vi "GUI_PI_Stages.vi"() -> ()   [LabVIEW 2013]
uses:
  <vilib>/Utility/tcp.llb/UDP Multicast Write-Only Open.vi
  <vilib>/Utility/file.llb/Read From Spreadsheet File (string).vi
panel:
  in  "QuadPosXYZ 2":dbl[](array[numeric])=[-4.0, 0.604, -0.05]
  out "Q2 controls":refnum<vi>[](array[refnum])
  out "Q1 controls":refnum<vi>[](array[refnum])
  out "DataSocket\nconnected":bool=TRUE
  out "QuadPosXYZ":dbl[](array[numeric])=[2.95001, 1.21, 2.60006, 2.57018, 2.80001, 11.9001]
  in  "Device Name 2":string="QuadZ"
  in  "Device Name":string="QuadXY"
  out "shotnumber":i32=-1
  out "con ref array":refnum<vi>[](array[refnum])
  out "MC Multicast":refnum<k16>
  out "new Slow Data":bool
  out "new Device Data":bool
  in  "Tab Control":T1(tab)
  out "limit Z2 (-)":dbl=-4.19999 format="%#_6f"
  out "limit Z1 (-)":dbl=-2.0 format="%#_6f"
  out "limit Z2 (+)":dbl=17.1 format="%#_6f"
  out "limit Z1 (+)":dbl=18.900100000000002 format="%#_6f"
  out "Z1":dbl=2.80001 format="%#_6f"
  in  "Q2 Z+":bool
  in  "Q2 Z-":bool
  out "Z2":dbl=11.9001 format="%#_6f"
  in  "Q1 Z+":bool
  in  "Q1 Z-":bool
  in  "Q2 Y+":bool
  in  "Q2 Y-":bool
  in  "Q2 X+":bool
  in  "Q2 X-":bool
  in  "Q1 Y-":bool
  in  "Q1 X+":bool
  in  "Q1 X-":bool
  in  "halt!":bool
  out "Y1":dbl=2.60006 format="%#_6f"
  out "Y2":dbl=2.57018 format="%#_6f"
  out "X1":dbl=2.95001 format="%#_6f"
  out "X2":dbl=1.21 format="%#_6f"
  out "error message":string
  out "error":bool
  in  "moving1":bool
  in  "moving2":bool
  in  "moving3":bool
  in  "moving4":bool
  out "Moving":bool
  out "Moving":bool
  in  "neglimit 1":bool
  in  "neglimit 2":bool
  in  "neglimit 3":bool
  in  "neglimit 4":bool
  in  "poslimit 1":bool
  in  "poslimit 3":bool
  in  "poslimit 4":bool
  in  "poslimit 2":bool
  in  "Q1 Y+":bool
  in  "Moving":bool
  in  "Moving":bool
  in  "poslimit 6":bool
  in  "neglimit 6":bool
  in  "poslimit 5":bool
  in  "neglimit 5":bool
  in  "servostatus 6":bool
  in  "servostatus 5":bool
  in  "servostatus 4":bool
  in  "servostatus 2":bool
  in  "servostatus 3":bool
  in  "servostatus 1":bool
  in  "save mode 2":bool=TRUE
  in  "save mode 3":bool=TRUE
  in  "setSaveMode":bool=TRUE
  in  "StepSize":dbl=1.5 format="%#_6f"
  out "data con closed":bool=TRUE
  out "data\nconnection 2":bool
  out "data con closed 2":bool=TRUE
  out "data\nconnection 3":bool
  out "Hexapos (Z)":dbl=-4.0
  out "D1":dbl=37.000009999999996 format="%#_6f"
  out "D2":dbl=24.70009 format="%#_6f"
  out "In Range?":bool=TRUE
  out "In Range?":bool=TRUE
  in  "Remote Host 2":string="192.168.10.75"
  in  "port or service name 2":u16=65534
  out "local Port":u16=65000
  out "Remote Host":string="192.168.10.73"
  out "port or service name":u16=65535
  in  "timeout ms (100)":i32=20
  in  "Multicast":bool
  out "#shot":i32
  in  "String 2":string
  in  "send CMD":bool
  in  "reset":bool
  in  "New Shot":bool
  in  "Data String 2":string="scalar>>pos2,2.800010\r\npos4,11.900100\r\nmoving2,off\r\nmoving4,off\r\ncloseaftermove,on\r\nservostatus2,off\r\nservostatus4,off\r\nneglimit2,off\r\nneglimit4,off\r\nposlimit2,off\r\nposlimit4,off\r\n"
  out "fast ID":refnum<k16>
  out "slow ID":refnum<k16>
  out "data connection ID":refnum<k5>
  out "connections":variant[](array[variant])=[variant(refnum<k16> refnum), variant(refnum<k16> refnum)]
  in  "time to wait":i32=25
  in  "Subscriber list 2":string="wait>>pos1,pos2,pos3,pos4,moving1,moving2,moving3,moving4,closeaftermove,servostatus1,servostatus2,servostatus3,servostatus4,neglimit1,neglimit2,neglimit3,neglimit4,poslimit1,poslimit2,poslimit3,poslimit4"
  in  "Data String":string="scalar>>pos1,2.950010\r\npos2,1.210000\r\npos3,2.600060\r\npos4,2.570180\r\nmoving1,off\r\nmoving2,off\r\nmoving3,off\r\nmoving4,off\r\ncloseaftermove,on\r\nservostatus1,off\r\nservostatus2,off\r\nservostatus3,off\r\nservostatus4,off\r\nneglimit1,off\r\nneglimit2,off\r\nneglimit3,off\r\nneglimit4,off\r\nposlimit1,off\r\nposlimit2,off\r\nposlimit3,off\r\nposlimit4,off\r\n"
  out "data connection ID 2":refnum<k5>
  in  "Subscriber list 3":string="wait>>pos2,pos4,moving2,moving4,closeaftermove,servostatus2,servostatus4,neglimit2,neglimit4,poslimit2,poslimit4"
  out "all rows":string[][](array[string])=[["localport", "65000"], ["port", "65535"], ["remotehost", "192.168.10.73"]]
  out "path":path=path "X:/Software/LOASIS Control System/Developers Version/Interface/GUI_PI_Stages/192.168.10.157.txt"
  out "My IP":string="192.168.10.157"
  out "error out":errorcluster
  in  "stop":bool
  # "QUAD 1"
  # "QUAD 2"
  # "connected"
  # "connected"
  # "Servo \nStatus"
  # "XY"
  # "Z"
  # "61525"
  # "65535"
  # "61533"
  # "localhost"
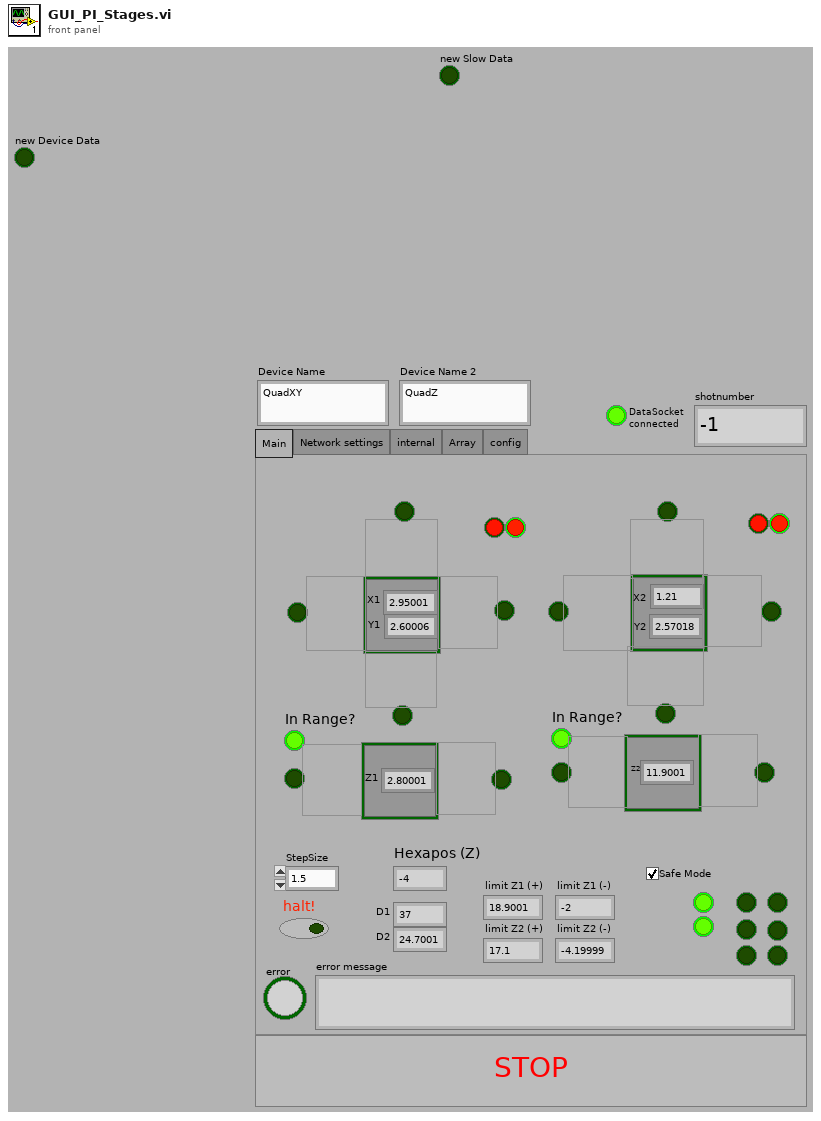
[diagram p1: front panel]
types:
  T1 = enum32{"Main", "Network settings", "internal", "Array", "config"}
  T2 = typedef "LVDataSocketStatusTypeDef.ctl" = cluster{"Code":enum32{"Invalid Status", "Unconnected", "Active", "Idle", "Error", "Connecting"}, "Text":string}
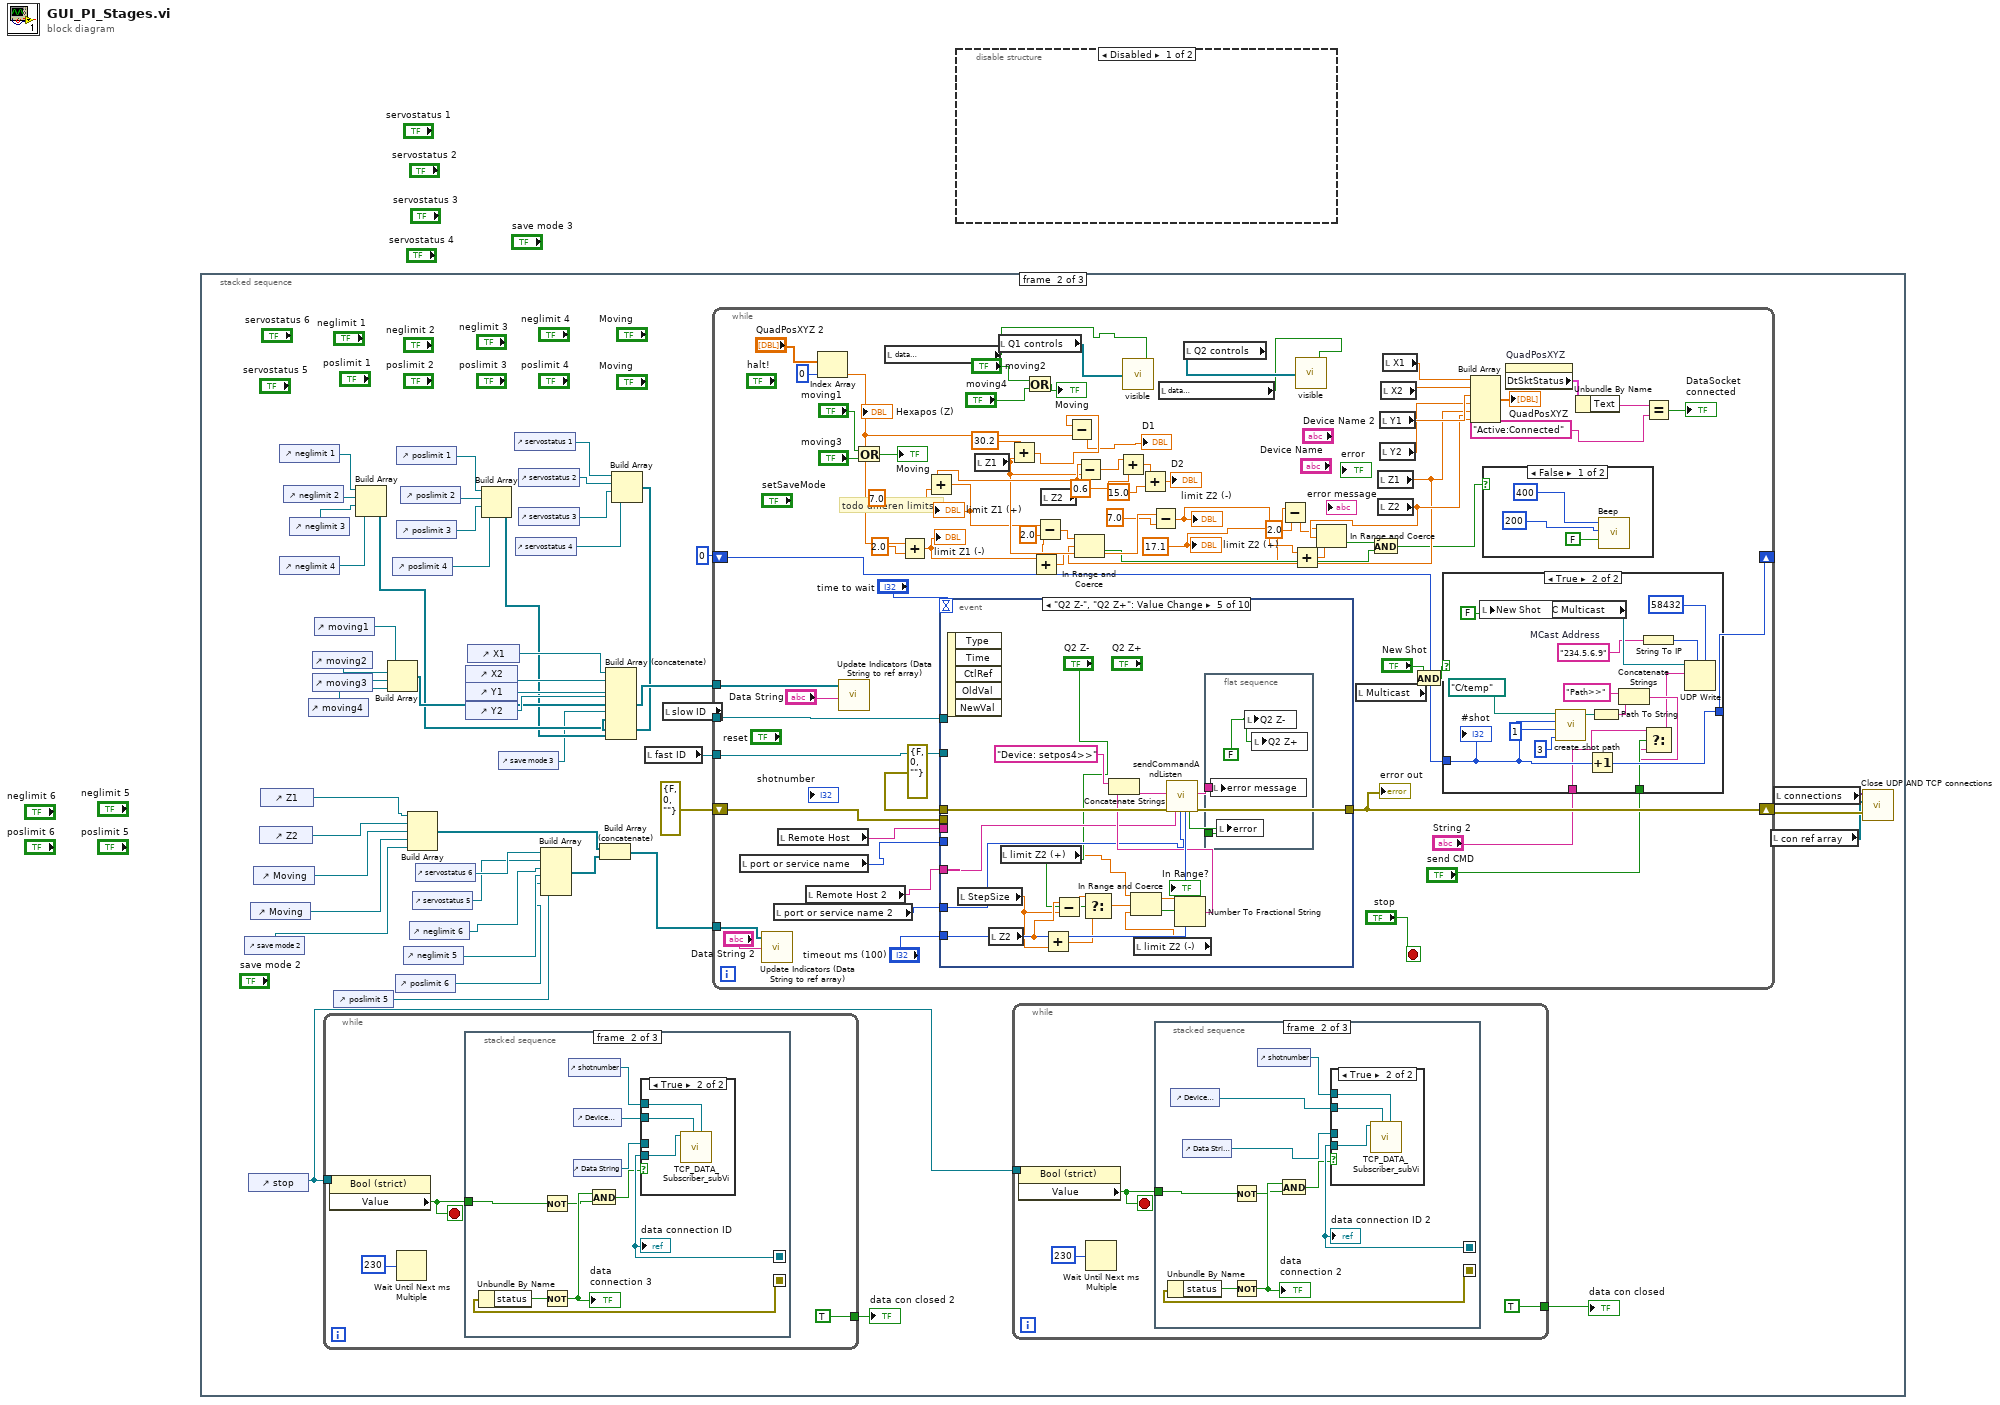
[diagram p0: block diagram]
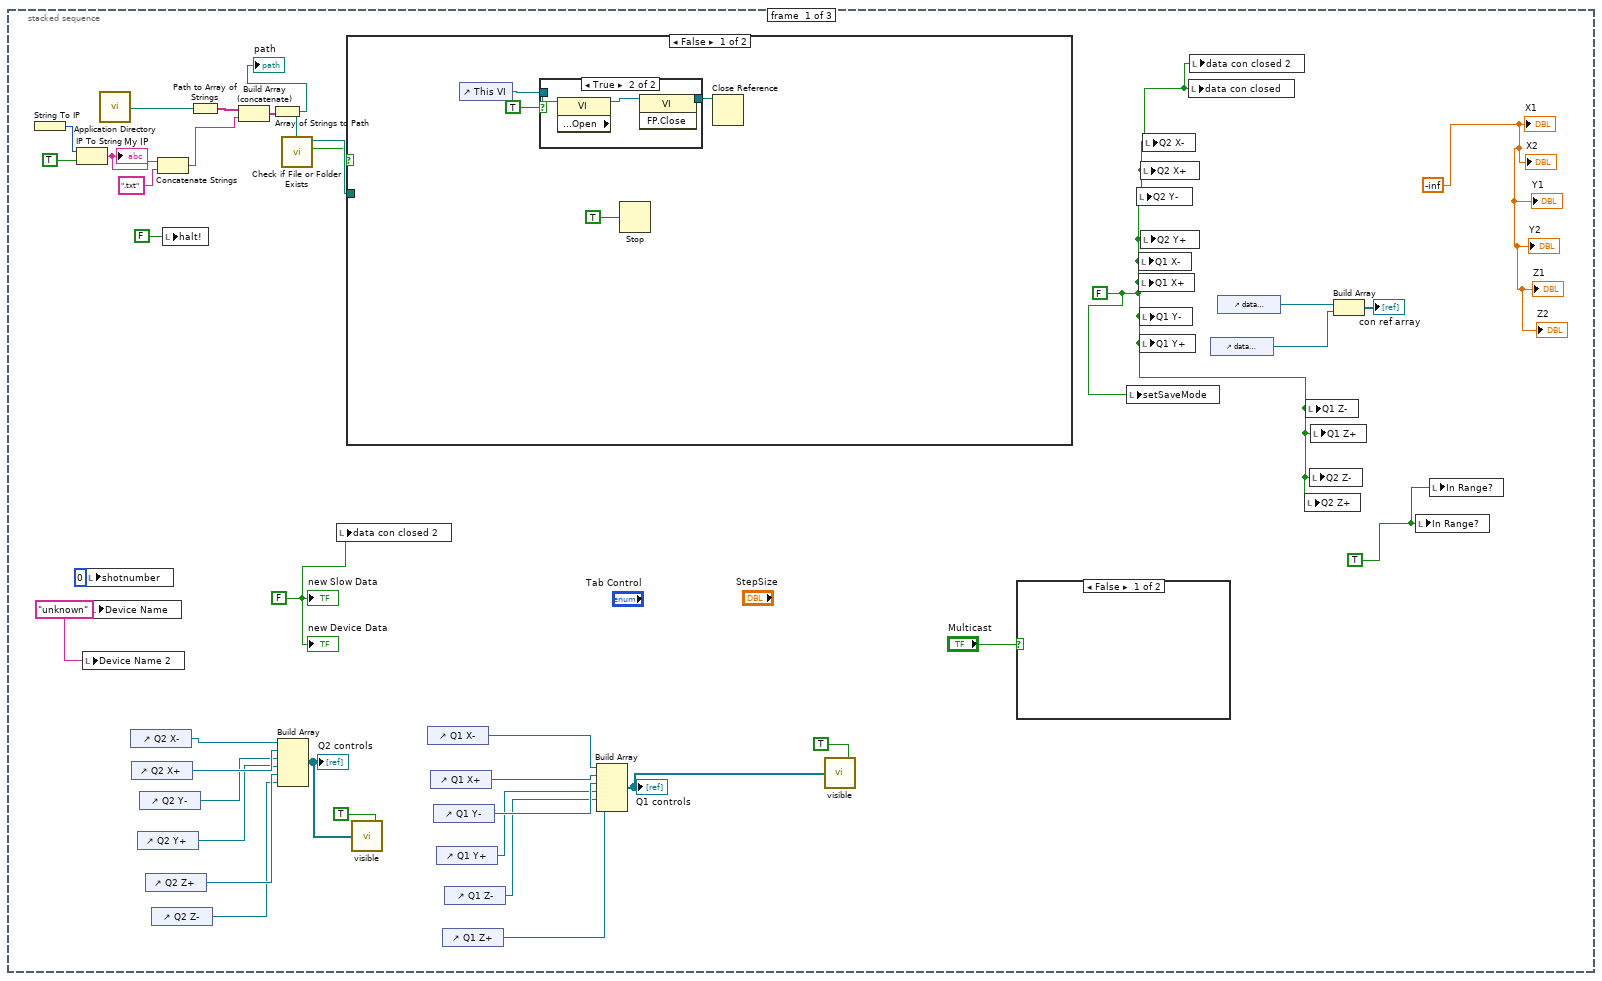
[diagram p3: hidden frame]
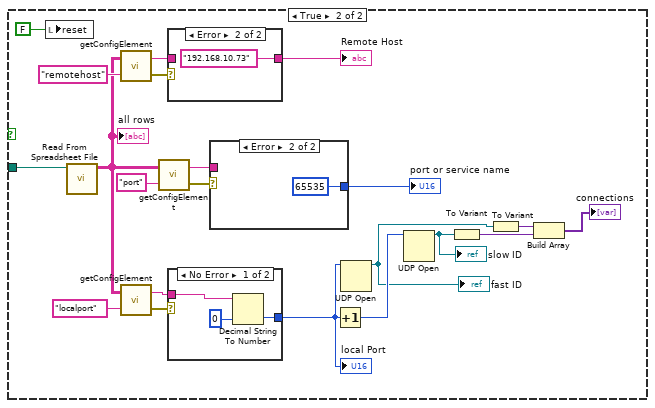
[diagram p5: hidden frame]
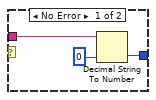
[diagram p6: hidden frame]
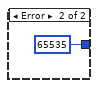
[diagram p8: hidden frame]
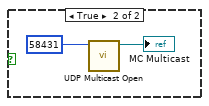
[diagram p9: hidden frame]
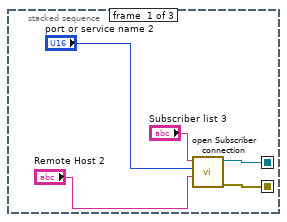
[diagram p10: hidden frame]
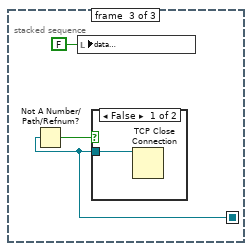
[diagram p12: hidden frame]
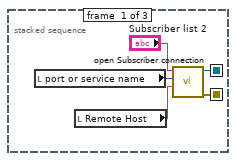
[diagram p14: hidden frame]
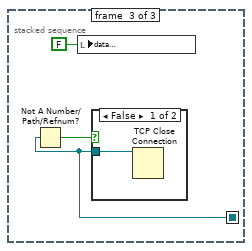
[diagram p16: hidden frame]
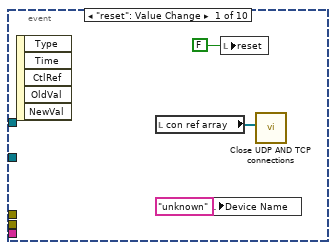
[diagram p20: hidden frame]
diagram:
  n1 = stacked-sequence {
    frame #0 {
      w1 = TRUE ("Q1 X-")
      w19 = -inf
      w18 = FALSE ("Q1 X-")
      w20 = "unknown" ("Device Name")
      w23 = FALSE ("new Device Data")
      n2 = String To IP() -> (0:w32:u32)  [unwired: 1 in]
      n3 = IP To String(1:TRUE ("dot notation? (F)"), 2:w32) -> (0:w30:string)
      "My IP" <- w30
      n4 = local write "Device Name 2"(w20) -> ()
      n5 = local write "shotnumber"(0 ("shotnumber")) -> ()
      n6 = local write "Device Name"(w20) -> ()
      n7 = call <vilib>:"Application Directory.vi"() -> ("Application Directory"=w28:path)
      n8 = control-ref of="Q2 X-"() -> (w17:refnum<vi>)
      n9 = control-ref of="Q2 X+"() -> (w16:refnum<vi>)
      n10 = control-ref of="Q2 Y+"() -> (w14:refnum<vi>)
      n11 = control-ref of="Q2 Y-"() -> (w15:refnum<vi>)
      n12 = control-ref of="Q2 Z+"() -> (w13:refnum<vi>)
      n13 = control-ref of="Q2 Z-"() -> (w12:refnum<vi>)
      n14 = Concatenate Strings(w30, ".txt" ("pattern")) -> (w27:string)
      n15 = local write "halt!"(FALSE ("halt!")) -> ()
      n16 = Path to Array of Strings(0:w28) -> (2:w34:string[])  [unwired: 1 out]
      n17 = Build Array (concatenate)(w34, w27) -> (w33:string[])
      n18 = Array of Strings to Path(0:w33) -> (2:w26:path)  [unwired: 1 in]
      "path" <- w26
      n19 = Build Array(w17, w16, w15, w14, w13, w12) -> (w3:refnum<vi>[])
      "Q2 controls" <- w3
      n20 = call <vilib>:"Check if File or Folder Exists.vi"("path"=w26) -> ("file or folder exists?"=w24:bool, "dup path"=w25:path)  [unwired: 8 in, 1 out]
      n21 = local write "data con closed 2"(w23) -> ()
      n22 = case shown="False" w24 {
        tunnel: w25 -> [_ w49]
        frame False {
          n23 = control-ref of="This VI"() -> (w41:refnum<vi>)
          n24 = case shown="True" TRUE {
            tunnel: w41 -> [w43 w46]
            tunnel: [w43 w44] -> w40
            frame False {
            }
            frame True {
              n25 = property class="VI" props=["Front Panel.Open"](reference=w46) -> (reference out=w45:refnum<vi>)  [unwired: 1 in, 2 out]
              n26 = invoke class="VI" method="FP.Close"(reference=w45) -> (reference out=w44:refnum<vi>)  [unwired: 2 in, 2 out]
            }
          }
          n27 = Stop(stop? (T)=TRUE) -> ()
          n28 = Close Reference(reference=w40) -> ()  [unwired: 1 in, 1 out]
        }
        frame True {
          n29 = local write "reset"(FALSE ("reset")) -> ()
          n30 = call-poly <vilib>:"Read From Spreadsheet File.vi"("file path (dialog if empty)"=w49) -> ("all rows"=w51:string[][])  [unwired: 6 in, 4 out]
          "all rows" <- w51
          n31 = call "getConfigElement.vi"("element"="remotehost", "all rows"=w51) -> ("error in"=w48:errorcluster, "value"=w56:string)
          n32 = call "getConfigElement.vi"("element"="localport", "all rows"=w51) -> ("error in"=w58:errorcluster, "value"=w59:string)
          n33 = call "getConfigElement.vi"("element"="port", "all rows"=w51) -> ("error in"=w47:errorcluster, "value"=w53:string)
          n34 = case shown="Error" w48 {
            tunnel: w56 -> [w72 _]
            tunnel: [w72 "192.168.10.73" ("value")] -> w54
            frame No Error {
            }
            frame Error {
            }
          }
          "Remote Host" <- w54
          n35 = case shown="No Error" w58 {
            tunnel: w59 -> [w76 _]
            tunnel: [w74 u16 65535] -> w57
            frame No Error {
              n36 = Decimal String To Number(string=w76, default (0L)=u16 0 ("local Port")) -> (number=w74:u16)  [unwired: 1 in, 1 out]
            }
            frame Error {
            }
          }
          "local Port" <- w57
          n37 = case shown="Error" w47 {
            tunnel: w53 -> [w70 _]
            tunnel: [w68 u16 65535] -> w50
            frame No Error {
              n38 = Decimal String To Number(string=w70, default (0L)=u16 0 ("local Port")) -> (number=w68:u16)  [unwired: 1 in, 1 out]
            }
            frame Error {
            }
          }
          "port or service name" <- w50
          n39 = Increment(x=w57) -> (x+1=w67:u16)
          n40 = UDP Open(11:w57) -> (port=w65:refnum<k16>)  [unwired: 4 in, 2 out]
          "fast ID" <- w65
          n41 = UDP Open(11:w67) -> (port=w64:refnum<k16>)  [unwired: 4 in, 2 out]
          "slow ID" <- w64
          n42 = To Variant(anything=w64) -> (Variant=w62:variant)
          n43 = To Variant(anything=w65) -> (Variant=w63:variant)
          n44 = Build Array(w63, w62) -> (→"connections":variant[])
        }
      }
      n45 = call "visible.vi"("visible"=TRUE, "Array"=w3) -> ()
      n46 = control-ref of="Q1 X-"() -> (w11:refnum<vi>)
      n47 = control-ref of="Q1 X+"() -> (w10:refnum<vi>)
      n48 = control-ref of="Q1 Y-"() -> (w9:refnum<vi>)
      n49 = control-ref of="Q1 Y+"() -> (w8:refnum<vi>)
      n50 = control-ref of="Q1 Z+"() -> (w6:refnum<vi>)
      n51 = control-ref of="Q1 Z-"() -> (w7:refnum<vi>)
      n52 = Build Array(w11, w10, w9, w8, w7, w6) -> (w5:refnum<vi>[])
      "Q1 controls" <- w5
      n53 = call "visible.vi"("visible"=TRUE, "Array"=w5) -> ()
      n54 = case shown="False" "Multicast" {
        frame False {
        }
        frame True {
          n55 = call-poly <vilib>:"UDP Multicast Open.vi"("port"=u16 58431) -> ("connection ID"=→"MC Multicast":refnum<k16>)  [unwired: 9 in, 1 out]
        }
      }
      n56 = local write "setSaveMode"(w18) -> ()
      n57 = local write "Q2 Y-"(w18) -> ()
      n58 = local write "Q1 X-"(w18) -> ()
      n59 = local write "Q1 X+"(w18) -> ()
      n60 = local write "Q1 Y-"(w18) -> ()
      n61 = local write "Q1 Y+"(w18) -> ()
      n62 = local write "Q2 X+"(w18) -> ()
      n63 = local write "Q2 Y+"(w18) -> ()
      n64 = local write "Q2 X-"(w18) -> ()
      n65 = local write "data con closed"(w18) -> ()
      n66 = local write "data con closed 2"(w18) -> ()
      n67 = control-ref of="data connection ID 2"() -> (w21:refnum<vi>)
      n68 = control-ref of="data connection ID"() -> (w38:refnum<vi>)
      n69 = local write "Q2 Z+"(w18) -> ()
      n70 = local write "Q1 Z-"(w18) -> ()
      n71 = local write "Q2 Z-"(w18) -> ()
      n72 = local write "Q1 Z+"(w18) -> ()
      n73 = Build Array(w38, w21) -> (→"con ref array":refnum<vi>[])
      n74 = local write "In Range?"(w1) -> ()
      n75 = local write "In Range?"(w1) -> ()
      "new Device Data" <- w23
      "new Slow Data" <- w23
      "X1" <- w19
      "X2" <- w19
      "Y2" <- w19
      "Y1" <- w19
      "Z1" <- w19
      "Z2" <- w19
    }
    frame #1 {
      n76 = control-ref of="save mode 2"() -> (w90:refnum<vi>)
      n77 = control-ref of="stop"() -> (w96:refnum<vi>)
      n78 = control-ref of="Moving"() -> (w91:refnum<vi>)
      n79 = control-ref of="Moving"() -> (w92:refnum<vi>)
      n80 = control-ref of="Z2"() -> (w93:refnum<vi>)
      n81 = control-ref of="Z1"() -> (w94:refnum<vi>)
      n82 = control-ref of="neglimit 1"() -> (w107:refnum<vi>)
      n83 = control-ref of="neglimit 4"() -> (w104:refnum<vi>)
      n84 = control-ref of="neglimit 2"() -> (w106:refnum<vi>)
      n85 = control-ref of="neglimit 3"() -> (w105:refnum<vi>)
      n86 = control-ref of="moving4"() -> (w114:refnum<vi>)
      n87 = control-ref of="moving2"() -> (w116:refnum<vi>)
      n88 = control-ref of="moving3"() -> (w115:refnum<vi>)
      n89 = control-ref of="moving1"() -> (w117:refnum<vi>)
      n90 = while {
        tunnel: [TRUE] -> w97
        tunnel: w96 -> [w157]
        stop <- w156 stop-if-true
        n91 = property class="Bool (strict)"(reference=w157) -> ("Value"=w156:bool)  [unwired: 1 in, 2 out]
        n92 = Wait Until Next ms Multiple(millisecond multiple=u32 230) -> ()  [unwired: 1 out]
        n93 = stacked-sequence {
          seq-local: [w161 _ _] -> [_ w173 w179]
          seq-local: [w160 _ _] -> [_ w172 _]
          tunnel: w156 -> [_ w166 _]
          frame #0 {
            n94 = local read "port or service name"() -> (w163:u16)
            n95 = local read "Remote Host"() -> (w162:string)
            n96 = call "open Subscriber connection.vi"("Machine"=w162, "Port"=w163, "Subscriber list"="Subscriber list 2") -> ("error out"=w160:errorcluster, "connection ID"=w161:refnum<k5>)  [unwired: 3 in]
          }
          frame #1 {
            n97 = Unbundle By Name(w172) -> ("status"=w169:bool)
            n98 = Not(x=w166) -> (.not. x?=w167:bool)
            n99 = Not(x=w169) -> (.not. x?=w168:bool)
            "data\nconnection 3" <- w168
            n100 = control-ref of="shotnumber"() -> (w171:refnum<vi>)
            n101 = control-ref of="Device Name"() -> (w170:refnum<vi>)
            n102 = control-ref of="Data String"() -> (w174:refnum<vi>)
            n103 = And(x=w168, y=w167) -> (x .and. y?=w165:bool)
            n104 = case shown="True" w165 {
              tunnel: w174 -> [_ _]
              tunnel: w173 -> [_ w175]
              tunnel: w171 -> [_ w177]
              tunnel: w170 -> [_ w176]
              frame False {
              }
              frame True {
                n105 = call "TCP_DATA_Subscriber_subVi.vi"("shot number"=w177, "whatamI"=w176, "connection ID"=w175) -> ()  [unwired: 8 in, 1 out]
              }
            }
            "data connection ID" <- w173
          }
          frame #2 {
            n106 = Not A Number/Path/Refnum?(number/path/refnum=w179) -> (NaN/Path/Refnum?=w180:bool)
            n107 = local write "data\nconnection 3"(FALSE ("status 2")) -> ()
            n108 = case shown="False" w180 {
              tunnel: w179 -> [w181 _]
              frame False {
                n109 = TCP Close Connection(connection ID=w181) -> ()  [unwired: 2 in, 2 out]
              }
              frame True {
              }
            }
          }
        }
      }
      "data con closed 2" <- w97
      n110 = control-ref of="poslimit 5"() -> (w84:refnum<vi>)
      n111 = Build Array(w107, w106, w105, w104) -> (w99:refnum<vi>[])
      n112 = Build Array(w117, w116, w115, w114) -> (w113:refnum<vi>[])
      n113 = control-ref of="poslimit 4"() -> (w100:refnum<vi>)
      n114 = control-ref of="poslimit 6"() -> (w85:refnum<vi>)
      n115 = control-ref of="poslimit 1"() -> (w103:refnum<vi>)
      n116 = control-ref of="poslimit 3"() -> (w101:refnum<vi>)
      n117 = control-ref of="poslimit 2"() -> (w102:refnum<vi>)
      n118 = control-ref of="neglimit 5"() -> (w86:refnum<vi>)
      n119 = Build Array(w94, w93, w92, w91, w90) -> (w83:refnum<vi>[])
      n120 = control-ref of="neglimit 6"() -> (w87:refnum<vi>)
      n121 = control-ref of="servostatus 5"() -> (w88:refnum<vi>)
      n122 = control-ref of="servostatus 6"() -> (w89:refnum<vi>)
      n123 = control-ref of="X2"() -> (w120:refnum<vi>)
      n124 = control-ref of="Y1"() -> (w119:refnum<vi>)
      n125 = control-ref of="Y2"() -> (w118:refnum<vi>)
      n126 = control-ref of="X1"() -> (w126:refnum<vi>)
      n127 = Build Array(w103, w102, w101, w100) -> (w98:refnum<vi>[])
      n128 = control-ref of="save mode 3"() -> (w80:refnum<vi>)
      n129 = control-ref of="servostatus 1"() -> (w112:refnum<vi>)
      n130 = control-ref of="servostatus 4"() -> (w109:refnum<vi>)
      n131 = control-ref of="servostatus 2"() -> (w111:refnum<vi>)
      n132 = control-ref of="servostatus 3"() -> (w110:refnum<vi>)
      n133 = Build Array(w89, w88, w87, w86, w85, w84) -> (w82:refnum<vi>[])
      n134 = Build Array (concatenate)(w83, w82) -> (w81:refnum<vi>[])
      n135 = Build Array(w112, w111, w110, w109) -> (w108:refnum<vi>[])
      n136 = Build Array (concatenate)(w126, w120, w119, w118, w113, w80, w108, w99, w98) -> (w124:refnum<vi>[])
      n137 = local read "fast ID"() -> (w128:refnum<k16>)
      n138 = local read "slow ID"() -> (w127:refnum<k16>)
      n139 = while {
        tunnel: w128 -> [w246]
        shift-right: [w244] -> w125
        shift-left: errorcluster {"status"=FALSE, "code"=0, "source"=""} ("error out") -> [w250]
        tunnel: w127 -> [w238]
        tunnel: w124 -> [w252]
        shift-right: [w243] -> _
        shift-left: 0 -> [w242]
        tunnel: w81 -> [w228]
        stop <- "stop" stop-if-true
        w186 = 2.0 ("y")
        w190 = 2.0 ("y")
        w192 = 17.1 ("y")
        # "todo differen limits"
        n140 = local read "port or service name"() -> (w247:u16)
        n141 = call "Update Indicators (Data String to ref array).vi"("Data String"="Data String 2", "Array"=w228) -> ()  [unwired: 4 in]
        n142 = local read "port or service name 2"() -> (w226:u16)
        n143 = local read "Remote Host"() -> (w248:string)
        n144 = local read "Remote Host 2"() -> (w227:string)
        n145 = Index Array(array="QuadPosXYZ 2", index=0) -> (element=w201:dbl)
        "Hexapos (Z)" <- w201
        n146 = call "Update Indicators (Data String to ref array).vi"("Data String"="Data String", "Array"=w252) -> ()  [unwired: 4 in]
        n147 = Or(x="moving1", y="moving3") -> (x .or. y?=→"Moving":bool)
        n148 = local read "data\nconnection 3"() -> (w214:bool)
        n149 = Add(x=w201, y=2.0) -> (x+y=w191:dbl)
        "limit Z1 (-)" <- w191
        n150 = event shown="[4] \"Q2 Z-\", \"Q2 Z+\": Value Change" {
          selector: _ -> [_ _ _ _ _ _ _ _ _ _]
          dyn-events: _ -> [_ _ _ _ _ _ _ _ _ _]
          timeout: "time to wait" -> [_ _ _ _ _ _ _ _ _ _]
          tunnel: w246 -> [_ _ _ _ _ _ _ _ _ _]
          tunnel: [_ w291 w310 w333 w356 w375 w394 w405 w422 w431] -> w244
          tunnel: errorcluster {"status"=FALSE, "code"=0, "source"=""} ("error out") -> [_ w292 w311 w334 w357 w376 w395 w415 w422 _]
          tunnel: w248 -> [_ w290 w309 _ _ w374 w393 w414 w429 _]
          tunnel: w247 -> [_ w289 w308 _ _ w373 w392 w413 w428 _]
          tunnel: "timeout ms (100)" -> [_ w288 w307 w332 w355 w372 w391 w401 _ _]
          tunnel: w238 -> [_ _ _ _ _ _ _ _ _ _]
          tunnel: w250 -> [_ _ _ _ _ _ _ _ _ w431]
          tunnel: w227 -> [_ _ _ w323 w347 _ _ w403 w419 _]
          tunnel: w226 -> [_ _ _ w324 w348 _ _ w402 w418 _]
          event "reset": Value Change {
            n151 = event-data() -> ()  [unwired: 1 in, 5 out]
            n152 = local read "con ref array"() -> (w277:refnum<vi>[])
            n153 = local write "Device Name"("unknown" ("Device Name")) -> ()
            n154 = local write "reset"(FALSE ("reset")) -> ()
            n155 = call "Close UDP AND TCP connections.vi"("appended array 2"=w277) -> ()  [unwired: 7 in]
          }
          event "Q1 X-", "Q1 X+": Value Change {
            n156 = event-data() -> ()  [unwired: 1 in, 5 out]
            n157 = local read "StepSize"() -> (w279:dbl)
            n158 = local read "X1"() -> (w280:dbl)
            n159 = Add(x=w280, y=w279) -> (x+y=w283:dbl)
            n160 = Subtract(x=w280, y=w279) -> (x-y=w284:dbl)
            n161 = Select(t=w284, s="Q1 X-", f=w283) -> (s? t:f=w282:dbl)
            n162 = Number To Fractional String(number=w282) -> (F-format string=w281:string)  [unwired: 3 in]
            n163 = Concatenate Strings("Device: setpos1>>" ("data in"), w281) -> (w293:string)
            n164 = call "sendCommandAndListen.vi"("command in"=w293, "error in"=w292, "Remote Host"=w290, "port or service name"=w289, "timeout ms (100)"=w288) -> ("error"=w286:bool, "error message"=w287:string, "error out"=w291:errorcluster)  [unwired: 7 in, 5 out]
            n165 = flat-sequence {
              tunnel: w287 -> [w297]
              tunnel: w286 -> [w296]
              frame #0 {
                w295 = FALSE ("Q1 X-")
                n166 = local write "error message"(w297) -> ()
                n167 = local write "error"(w296) -> ()
                n168 = local write "Q1 X+"(w295) -> ()
                n169 = local write "Q1 X-"(w295) -> ()
              }
            }
          }
          event "Q1 Y-", "Q1 Y+": Value Change {
            n170 = event-data() -> ()  [unwired: 1 in, 5 out]
            n171 = local read "StepSize"() -> (w299:dbl)
            n172 = local read "Y1"() -> (w300:dbl)
            n173 = Add(x=w300, y=w299) -> (x+y=w303:dbl)
            n174 = Subtract(x=w300, y=w299) -> (x-y=w304:dbl)
            n175 = Select(t=w304, s="Q1 Y-", f=w303) -> (s? t:f=w302:dbl)
            n176 = Number To Fractional String(number=w302) -> (F-format string=w301:string)  [unwired: 3 in]
            n177 = Concatenate Strings("Device: setpos3>>" ("data in"), w301) -> (w312:string)
            n178 = call "sendCommandAndListen.vi"("command in"=w312, "error in"=w311, "Remote Host"=w309, "port or service name"=w308, "timeout ms (100)"=w307) -> ("error"=w305:bool, "error message"=w306:string, "error out"=w310:errorcluster)  [unwired: 7 in, 5 out]
            n179 = flat-sequence {
              tunnel: w306 -> [w316]
              tunnel: w305 -> [w315]
              frame #0 {
                w314 = FALSE ("Q1 X-")
                n180 = local write "error message"(w316) -> ()
                n181 = local write "error"(w315) -> ()
                n182 = local write "Q1 Y+"(w314) -> ()
                n183 = local write "Q1 Y-"(w314) -> ()
              }
            }
          }
          event "Q1 Z-", "Q1 Z+": Value Change {
            n184 = event-data() -> ()  [unwired: 1 in, 5 out]
            n185 = local read "StepSize"() -> (w319:dbl)
            n186 = local read "Z1"() -> (w326:dbl)
            n187 = local read "limit Z1 (+)"() -> (w318:dbl)
            n188 = Add(x=w326, y=w319) -> (x+y=w328:dbl)
            n189 = Subtract(x=w326, y=w319) -> (x-y=w329:dbl)
            n190 = local read "limit Z1 (-)"() -> (w317:dbl)
            n191 = Select(t=w329, s="Q1 Z-", f=w328) -> (s? t:f=w322:dbl)
            n192 = In Range and Coerce(upper limit=w318, x=w322, lower limit=w317) -> (coerced(x)=w321:dbl, In Range?=→"In Range?":bool)
            n193 = Number To Fractional String(number=w321) -> (F-format string=w327:string)  [unwired: 3 in]
            n194 = Concatenate Strings("Device: setpos2>>" ("data in"), w327) -> (w335:string)
            n195 = call "sendCommandAndListen.vi"("command in"=w335, "error in"=w334, "Remote Host"=w323, "port or service name"=w324, "timeout ms (100)"=w332) -> ("error"=w330:bool, "error message"=w331:string, "error out"=w333:errorcluster)  [unwired: 7 in, 5 out]
            n196 = flat-sequence {
              tunnel: w331 -> [w339]
              tunnel: w330 -> [w338]
              frame #0 {
                w337 = FALSE ("Q1 X-")
                n197 = local write "error message"(w339) -> ()
                n198 = local write "error"(w338) -> ()
                n199 = local write "Q1 Z-"(w337) -> ()
                n200 = local write "Q1 Z+"(w337) -> ()
              }
            }
          }
          event "Q2 Z-", "Q2 Z+": Value Change {
            n201 = event-data() -> ()  [unwired: 1 in, 5 out]
            n202 = local read "StepSize"() -> (w342:dbl)
            n203 = local read "Z2"() -> (w349:dbl)
            n204 = local read "limit Z2 (+)"() -> (w341:dbl)
            n205 = Add(x=w349, y=w342) -> (x+y=w351:dbl)
            n206 = Subtract(x=w349, y=w342) -> (x-y=w352:dbl)
            n207 = Select(t=w352, s="Q2 Z-", f=w351) -> (s? t:f=w344:dbl)
            n208 = local read "limit Z2 (-)"() -> (w340:dbl)
            n209 = In Range and Coerce(upper limit=w341, x=w344, lower limit=w340) -> (coerced(x)=w345:dbl, In Range?=→"In Range?":bool)
            n210 = Number To Fractional String(number=w345) -> (F-format string=w350:string)  [unwired: 3 in]
            n211 = Concatenate Strings("Device: setpos4>>" ("data in"), w350) -> (w358:string)
            n212 = call "sendCommandAndListen.vi"("command in"=w358, "error in"=w357, "Remote Host"=w347, "port or service name"=w348, "timeout ms (100)"=w355) -> ("error"=w353:bool, "error message"=w354:string, "error out"=w356:errorcluster)  [unwired: 7 in, 5 out]
            n213 = flat-sequence {
              tunnel: w354 -> [w362]
              tunnel: w353 -> [w361]
              frame #0 {
                w360 = FALSE ("Q1 X-")
                n214 = local write "error message"(w362) -> ()
                n215 = local write "error"(w361) -> ()
                n216 = local write "Q2 Z-"(w360) -> ()
                n217 = local write "Q2 Z+"(w360) -> ()
              }
            }
          }
          event "Q2 Y-", "Q2 Y+": Value Change {
            n218 = event-data() -> ()  [unwired: 1 in, 5 out]
            n219 = local read "StepSize"() -> (w364:dbl)
            n220 = local read "Y2"() -> (w365:dbl)
            n221 = Add(x=w365, y=w364) -> (x+y=w368:dbl)
            n222 = Subtract(x=w365, y=w364) -> (x-y=w369:dbl)
            n223 = Select(t=w369, s="Q2 Y-", f=w368) -> (s? t:f=w367:dbl)
            n224 = Number To Fractional String(number=w367) -> (F-format string=w366:string)  [unwired: 3 in]
            n225 = Concatenate Strings("Device: setpos4>>" ("data in"), w366) -> (w377:string)
            n226 = call "sendCommandAndListen.vi"("command in"=w377, "error in"=w376, "Remote Host"=w374, "port or service name"=w373, "timeout ms (100)"=w372) -> ("error"=w370:bool, "error message"=w371:string, "error out"=w375:errorcluster)  [unwired: 7 in, 5 out]
            n227 = flat-sequence {
              tunnel: w371 -> [w381]
              tunnel: w370 -> [w380]
              frame #0 {
                w379 = FALSE ("Q1 X-")
                n228 = local write "error message"(w381) -> ()
                n229 = local write "error"(w380) -> ()
                n230 = local write "Q2 Y-"(w379) -> ()
                n231 = local write "Q2 Y+"(w379) -> ()
              }
            }
          }
          event "Q2 X-", "Q2 X+": Value Change {
            n232 = event-data() -> ()  [unwired: 1 in, 5 out]
            n233 = local read "StepSize"() -> (w383:dbl)
            n234 = local read "X2"() -> (w384:dbl)
            n235 = Add(x=w384, y=w383) -> (x+y=w387:dbl)
            n236 = Subtract(x=w384, y=w383) -> (x-y=w388:dbl)
            n237 = Select(t=w388, s="Q2 X-", f=w387) -> (s? t:f=w386:dbl)
            n238 = Number To Fractional String(number=w386) -> (F-format string=w385:string)  [unwired: 3 in]
            n239 = Concatenate Strings("Device: setpos2>>" ("data in"), w385) -> (w396:string)
            n240 = call "sendCommandAndListen.vi"("command in"=w396, "error in"=w395, "Remote Host"=w393, "port or service name"=w392, "timeout ms (100)"=w391) -> ("error"=w389:bool, "error message"=w390:string, "error out"=w394:errorcluster)  [unwired: 7 in, 5 out]
            n241 = flat-sequence {
              tunnel: w390 -> [w400]
              tunnel: w389 -> [w399]
              frame #0 {
                w398 = FALSE ("Q1 X-")
                n242 = local write "error message"(w400) -> ()
                n243 = local write "error"(w399) -> ()
                n244 = local write "Q2 X+"(w398) -> ()
                n245 = local write "Q2 X-"(w398) -> ()
              }
            }
          }
          event "setSaveMode": Value Change {
            n246 = event-data() -> ("NewVal"=w410:bool)  [unwired: 1 in, 4 out]
            n247 = Select(t="on" ("data in"), s=w410, f="off" ("data in")) -> (s? t:f=w407:string)
            n248 = Concatenate Strings("Device: setcloseaftermove>>" ("data in"), w407) -> (w404:string)
            n249 = call "sendCommandAndListen.vi"("command in"=w404, "error in"=w415, "Remote Host"=w414, "port or service name"=w413, "timeout ms (100)"=w401) -> ("error"=w411:bool, "error message"=w412:string, "error out"=w406:errorcluster)  [unwired: 7 in, 5 out]
            n250 = local write "error message"(w412) -> ()
            n251 = local write "error"(w411) -> ()
            n252 = call "sendCommandAndListen.vi"("command in"=w404, "error in"=w406, "Remote Host"=w403, "port or service name"=w402, "timeout ms (100)"=w401) -> ("error out"=w405:errorcluster)  [unwired: 7 in, 7 out]
          }
          event "halt!": Value Change {
            w417 = 10 ("timeout ms (100)")
            n253 = event-data() -> ()  [unwired: 1 in, 5 out]
            n254 = Concatenate Strings("Device: sethalt>>" ("data in"), "on") -> (w423:string)
            n255 = call "sendCommandAndListen.vi"("command in"=w423, "Remote Host"=w429, "port or service name"=w428, "timeout ms (100)"=w417) -> ("error"=w426:bool, "error message"=w427:string, "error out"=w421:errorcluster)  [unwired: 8 in, 5 out]
            n256 = local write "halt!"(FALSE ("halt!")) -> ()
            n257 = local write "error message"(w427) -> ()
            n258 = local write "error"(w426) -> ()
            n259 = call "sendCommandAndListen.vi"("command in"=w423, "Remote Host"=w419, "port or service name"=w418, "timeout ms (100)"=w417) -> ("error out"=w420:errorcluster)  [unwired: 8 in, 7 out]
            n260 = call <vilib>:"Clear Errors.vi"("error in (no error)"=w421) -> ()  [unwired: 6 in, 1 out]
            n261 = call <vilib>:"Clear Errors.vi"("error in (no error)"=w420) -> ()  [unwired: 6 in, 1 out]
          }
          event Timeout {
            n262 = event-data() -> ()  [unwired: 1 in, 2 out]
          }
        }
        "error out" <- w244
        n263 = local read "Z1"() -> (w205:dbl)
        n264 = local read "Q1 controls"() -> (w216:refnum<vi>[])
        n265 = Add(x=30.2, y=w205) -> (x+y=w203:dbl)
        n266 = Or(x="moving2", y="moving4") -> (x .or. y?=→"Moving":bool)
        n267 = Add(x=w190, y=w191) -> (x+y=w189:dbl)
        n268 = local read "Z2"() -> (w207:dbl)
        n269 = Add(x=w207, y=7.0) -> (x+y=w194:dbl)
        "limit Z1 (+)" <- w194
        n270 = Subtract(x=w194, y=w190) -> (x-y=w193:dbl)
        n271 = Subtract(x=w203, y=w201) -> (x-y=→"D1":dbl)
        n272 = Subtract(x=w207, y=w205) -> (x-y=w184:dbl)
        n273 = Add(x=w184, y=0.6) -> (x+y=w182:dbl)
        n274 = call "visible.vi"("visible"=w214, "Array"=w216) -> ()
        n275 = Add(x=w182, y=15.0) -> (x+y=→"D2":dbl)
        n276 = Subtract(x=w205, y=7.0) -> (x-y=w187:dbl)
        "limit Z2 (-)" <- w187
        n277 = local read "data\nconnection 2"() -> (w213:bool)
        n278 = local read "Q2 controls"() -> (w215:refnum<vi>[])
        n279 = Subtract(x=w192, y=w186) -> (x-y=w188:dbl)
        n280 = Add(x=w187, y=w186) -> (x+y=w185:dbl)
        n281 = call "visible.vi"("visible"=w213, "Array"=w215) -> ()
        n282 = local read "Multicast"() -> (w241:bool)
        n283 = local read "Z1"() -> (w198:dbl)
        n284 = In Range and Coerce(upper limit=w193, x=w198, lower limit=w189) -> (In Range?=w196:bool)  [unwired: 1 out]
        n285 = local read "Z2"() -> (w199:dbl)
        n286 = In Range and Coerce(upper limit=w188, x=w199, lower limit=w185) -> (In Range?=w197:bool)  [unwired: 1 out]
        n287 = And(x=w197, y=w196) -> (x .and. y?=w195:bool)
        n288 = local read "Y1"() -> (w223:dbl)
        n289 = local read "Y2"() -> (w222:dbl)
        n290 = local read "X2"() -> (w224:dbl)
        n291 = local read "X1"() -> (w225:dbl)
        n292 = And(x="New Shot", y=w241) -> (x .and. y?=w239:bool)
        n293 = case shown="True" w239 {
          tunnel: w242 -> [w258 w264]
          tunnel: [w258 w263] -> w243
          tunnel: "send CMD" -> [_ w262]
          tunnel: "String 2" -> [_ w261]
          frame False {
          }
          frame True {
            w269 = "234.5.6.9"  # MCast Address
            n294 = local write "New Shot"(FALSE ("New Shot")) -> ()
            n295 = local read "MC Multicast"() -> (w270:refnum<k16>)
            n296 = call "create shot path.vi"("width (-)"=i16 3, "Shot Number"=w264, "Scan Number"=1, "Scans Path"=path "C:/temp") -> ("Device xxx path"=w273:path)  [unwired: 2 in]
            n297 = Increment(x=w264) -> (x+1=w263:i32)
            n298 = Path To String(path=w273) -> (string=w271:string)
            n299 = Concatenate Strings("Path>>" ("string"), w271) -> (w260:string)
            n300 = String To IP(1:w269) -> (0:w275:u32)
            n301 = Select(t=w261, s=w262, f=w260) -> (s? t:f=w259:string)
            n302 = UDP Write(address=w275, port or service name=u16 58432, connection ID=w270, data in=w259) -> ()  [unwired: 2 in, 2 out]
            "#shot" <- w264
          }
        }
        n303 = Build Array(w225, w224, w223, w222, w198, w199) -> (→"QuadPosXYZ":dbl[])
        n304 = case shown="False" w195 {
          frame False {
            n305 = call <vilib>:"Beep.vi"("use system alert? (T)"=FALSE, "duration (msec)"=u32 200, "frequency (Hz)"=u32 400) -> ()  [unwired: 9 in]
          }
          frame True {
          }
        }
        n306 = property on="QuadPosXYZ" class="Arr (strict)"() -> ("DtSktStatus"=w220:T2)  [unwired: 2 in, 2 out]
        n307 = Unbundle By Name(w220) -> ("Text"=w219:string)
        n308 = Equal?(x=w219, y="Active:Connected") -> (x = y?=→"DataSocket\nconnected":bool)
        "limit Z2 (+)" <- w192
      }
      n309 = while {
        tunnel: [TRUE] -> w95
        tunnel: w96 -> [w131]
        stop <- w130 stop-if-true
        n310 = property class="Bool (strict)"(reference=w131) -> ("Value"=w130:bool)  [unwired: 1 in, 2 out]
        n311 = Wait Until Next ms Multiple(millisecond multiple=u32 230) -> ()  [unwired: 1 out]
        n312 = stacked-sequence {
          seq-local: [w137 _ _] -> [_ w148 w153]
          seq-local: [w136 _ _] -> [_ w147 _]
          tunnel: w130 -> [_ w142 _]
          frame #0 {
            n313 = call "open Subscriber connection.vi"("Machine"="Remote Host 2", "Port"="port or service name 2", "Subscriber list"="Subscriber list 3") -> ("error out"=w136:errorcluster, "connection ID"=w137:refnum<k5>)  [unwired: 3 in]
          }
          frame #1 {
            n314 = Unbundle By Name(w147) -> ("status"=w145:bool)
            n315 = control-ref of="Device Name 2"() -> (w140:refnum<vi>)
            n316 = control-ref of="Data String 2"() -> (w139:refnum<vi>)
            n317 = Not(x=w142) -> (.not. x?=w143:bool)
            n318 = Not(x=w145) -> (.not. x?=w144:bool)
            "data\nconnection 2" <- w144
            n319 = control-ref of="shotnumber"() -> (w146:refnum<vi>)
            n320 = And(x=w144, y=w143) -> (x .and. y?=w141:bool)
            n321 = case shown="True" w141 {
              tunnel: w139 -> [_ _]
              tunnel: w148 -> [_ w151]
              tunnel: w146 -> [_ w150]
              tunnel: w140 -> [_ w149]
              frame False {
              }
              frame True {
                n322 = call "TCP_DATA_Subscriber_subVi.vi"("shot number"=w150, "whatamI"=w149, "connection ID"=w151) -> ()  [unwired: 8 in, 1 out]
              }
            }
            "data connection ID 2" <- w148
          }
          frame #2 {
            n323 = Not A Number/Path/Refnum?(number/path/refnum=w153) -> (NaN/Path/Refnum?=w154:bool)
            n324 = local write "data\nconnection 2"(FALSE ("status 2")) -> ()
            n325 = case shown="False" w154 {
              tunnel: w153 -> [w155 _]
              frame False {
                n326 = TCP Close Connection(connection ID=w155) -> ()  [unwired: 2 in, 2 out]
              }
              frame True {
              }
            }
          }
        }
      }
      "data con closed" <- w95
      n327 = local read "con ref array"() -> (w123:refnum<vi>[])
      n328 = local read "connections"() -> (w121:variant[])
      n329 = call "Close UDP AND TCP connections.vi"("error in"=w125, "appended array 2"=w123, "appended array"=w121) -> ()  [unwired: 5 in]
    }
    frame #2 {
      n330 = flat-sequence {
        frame #0 {
          n331 = Wait (ms)(milliseconds to wait=u32 0) -> ()  [unwired: 1 out]
        }
        frame #1 {
          n332 = local write "stop"(FALSE ("stop")) -> ()
        }
        frame #2 {
          n333 = control-ref of="This VI"() -> (w436:refnum<vi>)
          n334 = case shown="True" FALSE {
            tunnel: w436 -> [w437 w440]
            tunnel: [w437 w438] -> w435
            frame False {
            }
            frame True {
              n335 = property class="VI" props=["Front Panel.Open"](reference=w440) -> (reference out=w439:refnum<vi>)  [unwired: 1 in, 2 out]
              n336 = invoke class="VI" method="FP.Close"(reference=w439) -> (reference out=w438:refnum<vi>)  [unwired: 2 in, 2 out]
            }
          }
          n337 = Close Reference(reference=w435) -> ()  [unwired: 1 in, 1 out]
        }
      }
    }
  }
  n338 = disable-structure shown="Disabled" {
    frame Disabled {
    }
    frame Enabled {
    }
  }
